vi "SwerveDeadBand.vi"(1 "FrontRightRotationIn":dbl, 2 "FrontRightDriveIn":dbl, 5 "RearLeftRotationIn":dbl, 6 "RearLeftDriveIn":dbl, 8 "FrontLeftDriveIn":dbl, 9 "RearRightRotationIn":dbl, 12 "FrontLeftRotationIn":dbl, 13 "RearRightDriveIn":dbl, 17 "RotationSettings":T5={"T0"=0, "Mode"=enum."Home", "Rotation Neutral Mode"=enum."Override to Coast", "Rotation Control Mode"=0, "Feedback Device"=8} {"Rotation Control Mode" items=["PercentOutput"=0, "Position"=1, "Velocity"=2, "Current"=3, "Follower"=5, "MotionProfile"=6, "MotionMagic"=7, "MotionProfileArc"=10, "Disabled"=15]; "Feedback Device" items=["QuadEncoder"=0, "Analog"=2, "Tachometer"=4, "Pulse Width Encoded Position"=8, "Sensor Sum (S0 + S1)"=9, "Sensor Difference (D0 - D1)"=10, "Remote Source 0"=11, "Remote Source 1"=12, "Software Emulated"=15]}) -> (20 "FrontLeftRotationOut":dbl, 21 "FrontLeftDriveOut":dbl, 22 "FrontRightRotationOut":dbl, 23 "FrontRightDriveOut":dbl, 24 "RearLeftRotationOut":dbl, 25 "RearLeftDriveOut":dbl, 26 "RearRightRotationOut":dbl, 27 "RearRightDriveOut":dbl)   [LabVIEW 2018]
uses:
  SwerveRotationCalibrate.ctl
  <vilib>/Rock Robotics/WPI/ThirdParty/Phoenix-LabVIEW/Motor Controller/Controls/CTRE_Phoenix_MotorControl_NeutralMode.ctl
  <vilib>/Rock Robotics/WPI/ThirdParty/Phoenix-LabVIEW/Motor Controller/Controls/CTRE_Phoenix_MotorControl_ControlMode.ctl
  <vilib>/Rock Robotics/WPI/ThirdParty/Phoenix-LabVIEW/Motor Controller/Controls/CTRE_Phoenix_MotorControl_FeedbackDevice.ctl
  336eaeb9-7ccf-4ad5-a096-8914645c78cc.vi
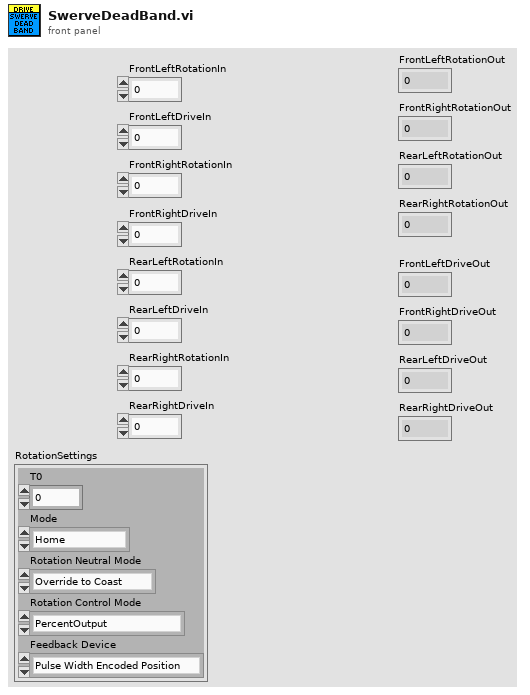
[diagram p1: front panel]
types:
  T1 = typedef "SwerveRotationCalibrate.ctl" = enum16{"Calibrate", "Home", "ResetQuad", "Drive"}
  T2 = typedef "CTRE_Phoenix_MotorControl_NeutralMode.ctl" = enum8{"EEPROMSetting", "Override to Coast", "Override to Brake"}
  T3 = typedef "CTRE_Phoenix_MotorControl_ControlMode.ctl" = u16
  T4 = typedef "CTRE_Phoenix_MotorControl_FeedbackDevice.ctl" = i8
  T5 = cluster{"T0":u32, "Mode":T1, "Rotation Neutral Mode":T2, "Rotation Control Mode":T3, "Feedback Device":T4}
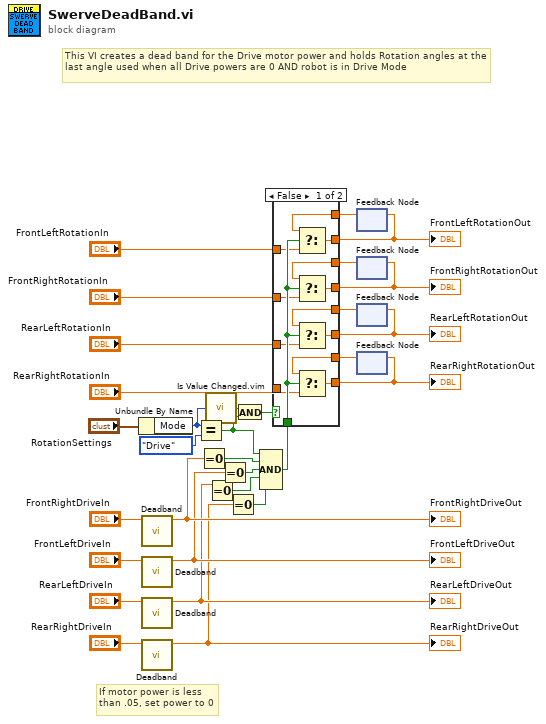
[diagram p0: block diagram]
diagram:
  # "This VI creates a dead band for the Drive motor power and holds Rotation angles at the last angle used when all Drive powers are 0 AND robot is in Drive Mode"
  # "If motor power is less than .05, set power to 0"
  n1 = Unbundle By Name("RotationSettings") -> ("Mode"=w8:T1)
  n2 = call "Deadband.vi"("Input"="FrontRightDriveIn") -> ("Output"=w26:dbl)  [unwired: 6 in]
  "FrontRightDriveOut" <- w26
  n3 = call "Deadband.vi"("Input"="FrontLeftDriveIn") -> ("Output"=w25:dbl)  [unwired: 6 in]
  "FrontLeftDriveOut" <- w25
  n4 = call "Deadband.vi"("Input"="RearLeftDriveIn") -> ("Output"=w23:dbl)  [unwired: 6 in]
  "RearLeftDriveOut" <- w23
  n5 = call "Deadband.vi"("Input"="RearRightDriveIn") -> ("Output"=w21:dbl)  [unwired: 6 in]
  "RearRightDriveOut" <- w21
  n6 = Equal?(x=w8, y=SwerveRotationCalibrate."Drive" ("x")) -> (x = y?=w7:bool)
  n7 = Equal To 0?(x=w26) -> (x = 0?=w10:bool)
  n8 = call "Is Value Changed.vim"("value"=w8) -> ("changed or first call?"=w6:bool)
  n9 = Equal To 0?(x=w23) -> (x = 0?=w22:bool)
  n10 = Equal To 0?(x=w25) -> (x = 0?=w24:bool)
  n11 = Equal To 0?(x=w21) -> (x = 0?=w20:bool)
  n12 = And(x=w6, y=w7) -> (x .and. y?=w1:bool)
  n13 = Compound Arithmetic op=AND(w7, w10, w24, w22, w20) -> (w27:bool)
  n14 = feedback #1() -> (w2:dbl)  [unwired: 1 in]
  n15 = feedback #2() -> (w3:dbl)  [unwired: 1 in]
  n16 = feedback #3() -> (w4:dbl)  [unwired: 1 in]
  n17 = feedback #4() -> (w5:dbl)  [unwired: 1 in]
  n18 = case shown="False" w1 {
    tunnel: w27 -> [w44 _]
    tunnel: "RearRightRotationIn" -> [w43 _]
    tunnel: "RearLeftRotationIn" -> [w42 _]
    tunnel: "FrontRightRotationIn" -> [w41 _]
    tunnel: "FrontLeftRotationIn" -> [w40 _]
    tunnel: [w39 _] -> w15
    tunnel: [w38 _] -> w14
    tunnel: [w37 _] -> w13
    tunnel: [w36 _] -> w12
    tunnel: w5 -> [w35 _]
    tunnel: w4 -> [w34 _]
    tunnel: w3 -> [w33 _]
    tunnel: w2 -> [w32 _]
    frame False {
      n19 = Select(t=w32, s=w44, f=w40) -> (s? t:f=w38:dbl)
      n20 = Select(t=w33, s=w44, f=w41) -> (s? t:f=w39:dbl)
      n21 = Select(t=w34, s=w44, f=w42) -> (s? t:f=w37:dbl)
      n22 = Select(t=w35, s=w44, f=w43) -> (s? t:f=w36:dbl)
    }
    frame True {
    }
  }
  "FrontLeftRotationOut" <- w14
  "FrontRightRotationOut" <- w15
  "RearLeftRotationOut" <- w13
  "RearRightRotationOut" <- w12
  n23 = feedback-in #1(w14) -> ()
  n24 = feedback-in #2(w15) -> ()
  n25 = feedback-in #3(w13) -> ()
  n26 = feedback-in #4(w12) -> ()
